vi "com_write_read.vi"(5 "2 nd Query?":bool, 6 "Query?":bool, 7 "error in":errorcluster, 9 "Command":string, 10 "VISA handle in":refnum<visa-resource-name>) -> (0 "error out":errorcluster, 1 "2nd Response":string, 2 "Response":string, 3 "VISA handle out":refnum<visa-resource-name>, 4 "TimeoutFlag":bool)   [LabVIEW 2014]
doc: "This VI allows to send a command to the controller SMC 100 and to receive a response via the connection RS232. It is used in each VI."
panel:
  out "String":string
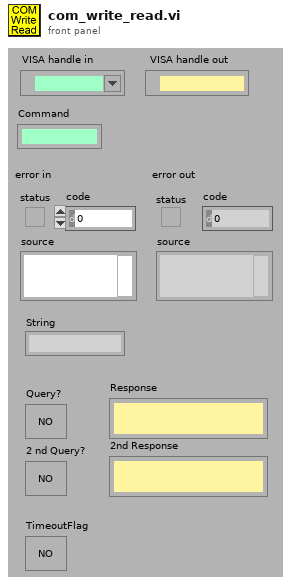
[diagram p1: front panel]
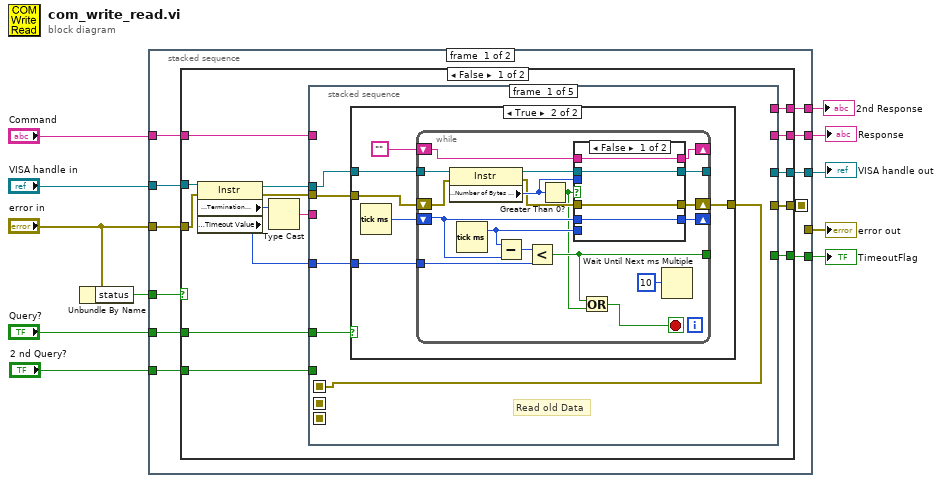
[diagram p0: block diagram]
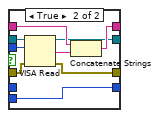
[diagram p3: hidden frame]
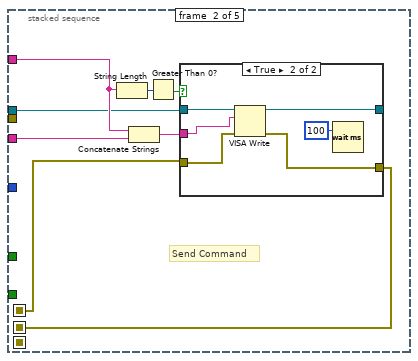
[diagram p4: hidden frame]
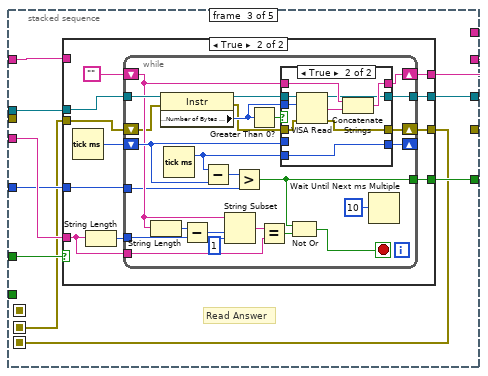
[diagram p6: hidden frame]
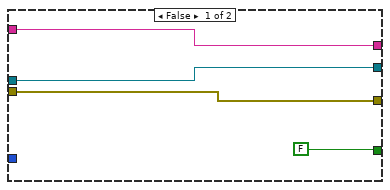
[diagram p7: hidden frame]
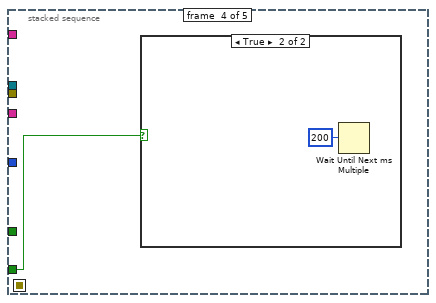
[diagram p9: hidden frame]
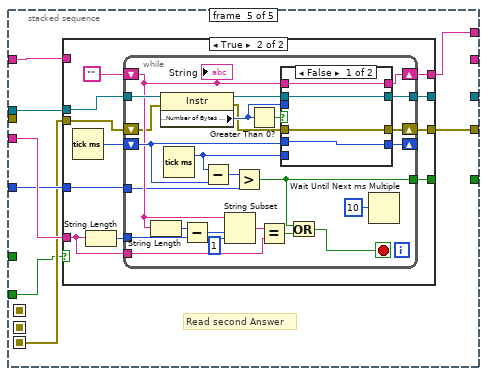
[diagram p11: hidden frame]
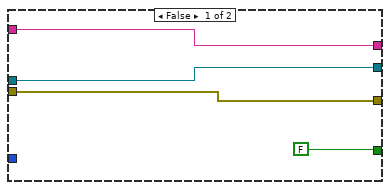
[diagram p12: hidden frame]
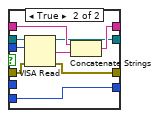
[diagram p13: hidden frame]
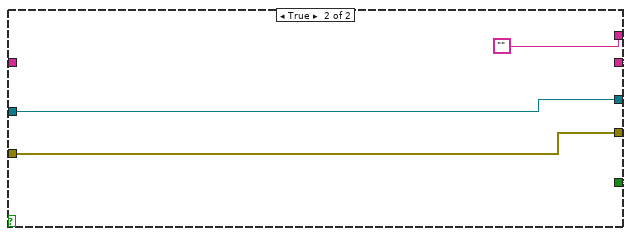
[diagram p14: hidden frame]
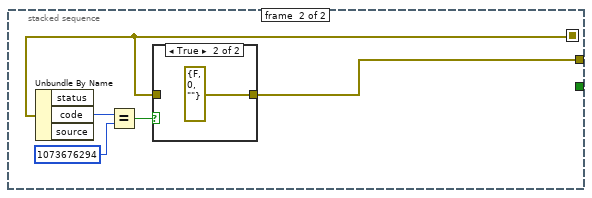
[diagram p15: hidden frame]
diagram:
  n1 = Unbundle By Name("error in") -> ("status"=w9:bool)
  n2 = stacked-sequence {
    seq-local: [w18 _] -> [_ w228]
    tunnel: "VISA handle in" -> [w22 _]
    tunnel: [_ w229] -> w10
    tunnel: w9 -> [w21 _]
    tunnel: "error in" -> [w20 _]
    tunnel: "Query?" -> [w19 _]
    tunnel: "Command" -> [w17 _]
    tunnel: [w16 _] -> w3
    tunnel: [w15 _] -> w5
    tunnel: [w14 _] -> w4
    tunnel: [w13 _] -> w2
    tunnel: "2 nd Query?" -> [w12 _]
    frame #0 {
      n3 = case shown="False" w21 {
        tunnel: w22 -> [w32 w227]
        tunnel: [w37 w227] -> w16
        tunnel: [w36 w226] -> w18
        tunnel: w20 -> [w29 w226]
        tunnel: [w35 ""] -> w14
        tunnel: [w34 FALSE] -> w15
        tunnel: w19 -> [w33 _]
        tunnel: w17 -> [w25 _]
        tunnel: [w24 ""] -> w13
        tunnel: w12 -> [w23 _]
        frame False {
          n4 = property class="Instr"(reference=w32, error in=w29) -> (reference out=w31:refnum<visa-resource-name>, error out=w28:errorcluster, "Message Based Settings:Termination Character"=w30:u8, "General Settings:Timeout Value"=w26:u32)
          n5 = Type Cast(x=w30) -> (*(type *) &x=w27:string)  [unwired: 1 in]
          n6 = stacked-sequence {
            seq-local: [w38 _ _ _ _] -> [_ w83 _ _ _]
            seq-local: [_ w81 _ _ _] -> [_ _ w98 _ _]
            seq-local: [_ _ w97 _ _] -> [_ _ _ _ w164]
            tunnel: [_ _ w106 _ _] -> w37
            tunnel: [_ _ _ _ w169] -> w36
            tunnel: [_ _ w100 _ _] -> w35
            tunnel: [_ _ w105 _ _] -> w34
            tunnel: w33 -> [w42 _ w104 _ _]
            tunnel: w31 -> [w40 w84 w99 _ w165]
            tunnel: w28 -> [w41 _ _ _ _]
            tunnel: w27 -> [_ w82 w103 _ w168]
            tunnel: w26 -> [w39 _ w102 _ w167]
            tunnel: w25 -> [_ w85 w101 _ w166]
            tunnel: [_ _ _ _ w163] -> w24
            tunnel: w23 -> [_ _ _ w160 w162]
            frame #0 {
              # "Read old Data"
              n7 = case shown="True" w42 {
                tunnel: [w43 w47] -> w38
                tunnel: w40 -> [_ w46]
                tunnel: w41 -> [w43 w45]
                tunnel: w39 -> [_ w44]
                frame False {
                }
                frame True {
                  n8 = Tick Count (ms)() -> (millisecond timer value=w49:u32)
                  n9 = while {
                    tunnel: w44 -> [w58]
                    tunnel: w46 -> [w67]
                    shift-right: [w64] -> _
                    shift-left: "" -> [w59]
                    shift-right: [w62] -> _
                    shift-left: w49 -> [w61]
                    tunnel: [w56] -> _
                    tunnel: [w55] -> _
                    shift-right: [w52] -> w47
                    shift-left: w45 -> [w54]
                    stop <- w57 stop-if-true
                    n10 = property class="Instr"(reference=w67, error in=w54) -> (reference out=w66:refnum<visa-resource-name>, error out=w53:errorcluster, "Serial Settings:Number of Bytes at Serial Port"=w65:u32)
                    n11 = Tick Count (ms)() -> (millisecond timer value=w63:u32)
                    n12 = Subtract(x=w63, y=w61) -> (x-y=w60:u32)
                    n13 = Less?(x=w60, y=w58) -> (x < y?=w56:bool)
                    n14 = Greater Than 0?(x=w65) -> (x > 0?=w50:bool)
                    n15 = case shown="False" w50 {
                      tunnel: w66 -> [w70 w80]
                      tunnel: w65 -> [_ w79]
                      tunnel: w59 -> [w71 w77]
                      tunnel: [w71 w76] -> w64
                      tunnel: w63 -> [_ w75]
                      tunnel: [w68 w75] -> w62
                      tunnel: w61 -> [w68 _]
                      tunnel: [w70 w74] -> w55
                      tunnel: w53 -> [w69 w73]
                      tunnel: [w69 w72] -> w52
                      frame False {
                      }
                      frame True {
                        n16 = VISA Read(VISA resource name=w80, byte count=w79, error in (no error)=w73) -> (VISA resource name out=w74:refnum<visa-resource-name>, read buffer=w78:string, error out=w72:errorcluster)  [unwired: 1 out]
                        n17 = Concatenate Strings(w77, w78) -> (w76:string)
                      }
                    }
                    n18 = Or(x=w56, y=w50) -> (x .or. y?=w57:bool)
                    n19 = Wait Until Next ms Multiple(millisecond multiple=u32 10) -> ()  [unwired: 1 out]
                  }
                }
              }
            }
            frame #1 {
              # "Send Command"
              n20 = String Length(string=w85) -> (length=w87:i32)
              n21 = Concatenate Strings(w85, w82) -> (w86:string)
              n22 = Greater Than 0?(x=w87) -> (x > 0?=w88:bool)
              n23 = case shown="True" w88 {
                tunnel: [w90 w96] -> _
                tunnel: [w89 w91] -> w81
                tunnel: w86 -> [_ w95]
                tunnel: w84 -> [w90 w94]
                tunnel: w83 -> [w89 w93]
                frame False {
                }
                frame True {
                  n24 = VISA Write(VISA resource name=w94, write buffer=w95, error in (no error)=w93) -> (VISA resource name out=w96:refnum<visa-resource-name>, error out=w91:errorcluster)  [unwired: 1 out]
                  n25 = Wait (ms)(milliseconds to wait=u32 100 ("Delay (ms)")) -> ()  [unwired: 1 out]
                }
              }
            }
            frame #2 {
              # "Read Answer"
              n26 = case shown="True" w104 {
                tunnel: [w109 w116] -> w97
                tunnel: [w110 w120] -> w106
                tunnel: w99 -> [w110 w112]
                tunnel: w98 -> [w109 w111]
                tunnel: [w107 w119] -> w100
                tunnel: [FALSE w117] -> w105
                tunnel: w101 -> [w107 _]
                tunnel: w103 -> [_ w114]
                tunnel: w102 -> [_ w113]
                frame False {
                }
                frame True {
                  n27 = Tick Count (ms)() -> (millisecond timer value=w121:u32)
                  n28 = String Length(string=w114) -> (length=w115:i32)
                  n29 = while {
                    tunnel: w115 -> [w125]
                    tunnel: w113 -> [w132]
                    tunnel: w112 -> [w146]
                    shift-right: [w142] -> w119
                    shift-left: "" -> [w133]
                    shift-right: [w140] -> _
                    shift-left: w121 -> [w139]
                    tunnel: w114 -> [w134]
                    tunnel: [w129] -> w117
                    tunnel: [w128] -> w120
                    shift-right: [w123] -> w116
                    shift-left: w111 -> [w127]
                    stop <- w130 stop-if-true
                    n30 = String Length(string=w133) -> (length=w137:i32)
                    n31 = property class="Instr"(reference=w146, error in=w127) -> (reference out=w144:refnum<visa-resource-name>, error out=w126:errorcluster, "Serial Settings:Number of Bytes at Serial Port"=w143:u32)
                    n32 = Tick Count (ms)() -> (millisecond timer value=w141:u32)
                    n33 = Subtract(x=w137, y=w125) -> (x-y=w136:i32)
                    n34 = Subtract(x=w141, y=w139) -> (x-y=w138:u32)
                    n35 = String Subset(string=w133, offset (0)=w136, length (rest)=1 ("longueur (reste)")) -> (substring=w135:string)
                    n36 = Greater?(x=w138, y=w132) -> (0:w129:bool)
                    n37 = Greater Than 0?(x=w143) -> (x > 0?=w145:bool)
                    n38 = Equal?(x=w135, y=w134) -> (x = y?=w131:bool)
                    n39 = case shown="True" w145 {
                      tunnel: w144 -> [w149 w159]
                      tunnel: w143 -> [_ w158]
                      tunnel: w133 -> [w150 w156]
                      tunnel: [w150 w155] -> w142
                      tunnel: w141 -> [_ w154]
                      tunnel: [w147 w154] -> w140
                      tunnel: w139 -> [w147 _]
                      tunnel: [w149 w153] -> w128
                      tunnel: w126 -> [w148 w152]
                      tunnel: [w148 w151] -> w123
                      frame False {
                      }
                      frame True {
                        n40 = VISA Read(VISA resource name=w159, byte count=w158, error in (no error)=w152) -> (VISA resource name out=w153:refnum<visa-resource-name>, read buffer=w157:string, error out=w151:errorcluster)  [unwired: 1 out]
                        n41 = Concatenate Strings(w156, w157) -> (w155:string)
                      }
                    }
                    n42 = Not Or(1:w131, 2:w129) -> (0:w130:bool)
                    n43 = Wait Until Next ms Multiple(millisecond multiple=u32 10) -> ()  [unwired: 1 out]
                  }
                }
              }
            }
            frame #3 {
              n44 = case shown="True" w160 {
                frame False {
                }
                frame True {
                  n45 = Wait Until Next ms Multiple(millisecond multiple=u32 200) -> ()  [unwired: 1 out]
                }
              }
            }
            frame #4 {
              # "Read second Answer"
              n46 = case shown="True" w162 {
                tunnel: [w172 w179] -> w169
                tunnel: [w173 w183] -> _
                tunnel: w165 -> [w173 w175]
                tunnel: w164 -> [w172 w174]
                tunnel: [w170 w182] -> w163
                tunnel: [FALSE w180] -> _
                tunnel: w166 -> [w170 _]
                tunnel: w168 -> [_ w177]
                tunnel: w167 -> [_ w176]
                frame False {
                }
                frame True {
                  n47 = Tick Count (ms)() -> (millisecond timer value=w184:u32)
                  n48 = String Length(string=w177) -> (length=w178:i32)
                  n49 = while {
                    tunnel: w178 -> [w188]
                    tunnel: w176 -> [w195]
                    tunnel: w175 -> [w209]
                    shift-right: [w205] -> w182
                    shift-left: "" -> [w196]
                    shift-right: [w203] -> _
                    shift-left: w184 -> [w202]
                    tunnel: w177 -> [w197]
                    tunnel: [w192] -> w180
                    tunnel: [w191] -> w183
                    shift-right: [w186] -> w179
                    shift-left: w174 -> [w190]
                    stop <- w193 stop-if-true
                    n50 = String Length(string=w196) -> (length=w200:i32)
                    n51 = property class="Instr"(reference=w209, error in=w190) -> (reference out=w207:refnum<visa-resource-name>, error out=w189:errorcluster, "Serial Settings:Number of Bytes at Serial Port"=w206:u32)
                    n52 = Tick Count (ms)() -> (millisecond timer value=w204:u32)
                    n53 = Subtract(x=w200, y=w188) -> (x-y=w199:i32)
                    n54 = Subtract(x=w204, y=w202) -> (x-y=w201:u32)
                    n55 = String Subset(string=w196, offset (0)=w199, length (rest)=1 ("longueur (reste)")) -> (substring=w198:string)
                    n56 = Greater?(x=w201, y=w195) -> (0:w192:bool)
                    n57 = Greater Than 0?(x=w206) -> (x > 0?=w208:bool)
                    n58 = Equal?(x=w198, y=w197) -> (x = y?=w194:bool)
                    n59 = case shown="False" w208 {
                      tunnel: w207 -> [w212 w222]
                      tunnel: w206 -> [_ w221]
                      tunnel: w196 -> [w213 w219]
                      tunnel: [w213 w218] -> w205
                      tunnel: w204 -> [_ w217]
                      tunnel: [w210 w217] -> w203
                      tunnel: w202 -> [w210 _]
                      tunnel: [w212 w216] -> w191
                      tunnel: w189 -> [w211 w215]
                      tunnel: [w211 w214] -> w186
                      frame False {
                      }
                      frame True {
                        n60 = VISA Read(VISA resource name=w222, byte count=w221, error in (no error)=w215) -> (VISA resource name out=w216:refnum<visa-resource-name>, read buffer=w220:string, error out=w214:errorcluster)  [unwired: 1 out]
                        n61 = Concatenate Strings(w219, w220) -> (w218:string)
                      }
                    }
                    n62 = Or(x=w192, y=w194) -> (x .or. y?=w193:bool)
                    n63 = Wait Until Next ms Multiple(millisecond multiple=u32 10) -> ()  [unwired: 1 out]
                    "String" <- w196
                  }
                }
              }
            }
          }
        }
        frame True {
        }
      }
    }
    frame #1 {
      n64 = Unbundle By Name(w228) -> ("code"=w232:i32)  [unwired: 2 out]
      n65 = Equal?(x=w232, y=1073676294) -> (x = y?=w231:bool)
      n66 = case shown="True" w231 {
        tunnel: w228 -> [w233 _]
        tunnel: [w233 errorcluster {"status"=FALSE, "code"=0, "source"=""} ("sortie d'erreur 2")] -> w229
        frame False {
        }
        frame True {
        }
      }
    }
  }
  "VISA handle out" <- w3
  "error out" <- w10
  "Response" <- w4
  "TimeoutFlag" <- w5
  "2nd Response" <- w2
